vi "NF LI56xx sub init data.vi"(8 "error in":errorcluster caption="error in (no error)" {"code" format="%.0x"}, 11 "VISA resource name":refnum<visa-resource-name>) -> (0 "error out":errorcluster {"code" format="%.0x"}, 3 "VISA resource name copy":refnum<visa-resource-name>)   [LabVIEW 2019]
doc: "get DATA parameters"
panel:
  out "DATA Out Cluster":T1
  in  "DATA Cluster":T1
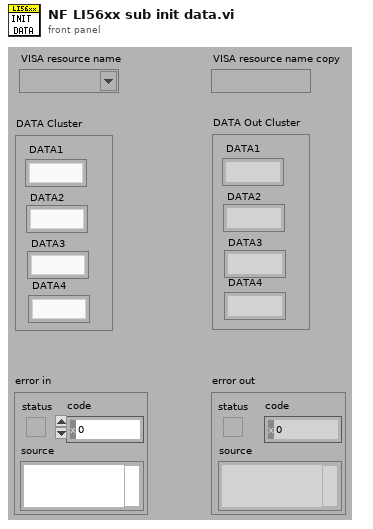
[diagram p1: front panel]
types:
  T1 = cluster{"DATA1":string, "DATA2":string, "DATA3":string, "DATA4":string}
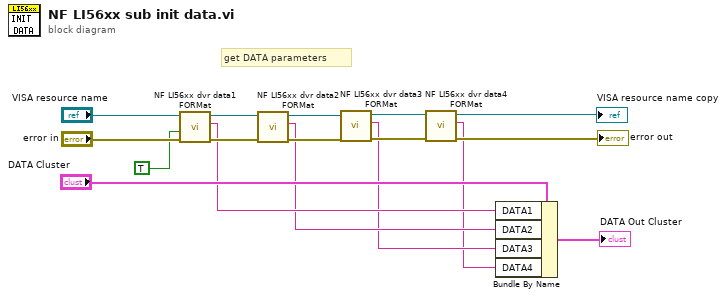
[diagram p0: block diagram]
diagram:
  # "get DATA parameters"
  n1 = call "NF LI56xx dvr data1 FORMat.vi"("error in"="error in", "Read(F)"=TRUE, "VISA resource name"="VISA resource name") -> ("error out"=w13:errorcluster, "query measurement \nparameters format"=w4:string, "VISA resource name copy"=w14:refnum<visa-resource-name>)  [unwired: 6 in]
  n2 = call "NF LI56xx dvr data2 FORMat.vi"("error in"=w13, "VISA resource name"=w14) -> ("error out"=w11:errorcluster, "query measurement\nparameters format"=w3:string, "VISA resource name copy"=w12:refnum<visa-resource-name>)  [unwired: 7 in]
  n3 = call "NF LI56xx dvr data3 FORMat.vi"("error in"=w11, "VISA resource name"=w12) -> ("error out"=w9:errorcluster, "query measurement \nparameters format"=w2:string, "VISA resource name copy"=w10:refnum<visa-resource-name>)  [unwired: 7 in]
  n4 = call "NF LI56xx dvr data4 FORMat.vi"("error in"=w9, "VISA resource name"=w10) -> ("error out"=→"error out":errorcluster, "query measurement \nparameters format"=w1:string, "VISA resource name copy"=→"VISA resource name copy":refnum<visa-resource-name>)  [unwired: 7 in]
  n5 = Bundle By Name(cluster="DATA Cluster", "DATA1"=w4, "DATA2"=w3, "DATA3"=w2, "DATA4"=w1) -> (→"DATA Out Cluster":T1)
